vi "SetRotation.vi"(7 "Relative?":bool, 8 "error in (no error)":errorcluster, 9 "Angle":sgl, 10 "Axis":cluster{"X":sgl, "Y":sgl, "Z":sgl}={"X"=0.0, "Y"=1.0, "Z"=0.0}, 11 "3D Object in":refnum<class "3D Object.lvclass">) -> (0 "error out":errorcluster, 3 "3D Object out":refnum<class "3D Object.lvclass">)   [LabVIEW 2015, in "3D Object.lvclass"]
uses:
  3D Object.lvclass
  3D Object.lvclass/3D Object.ctl
  <vilib>/picture/3D Picture Control/NI_3D Picture Control.lvlib
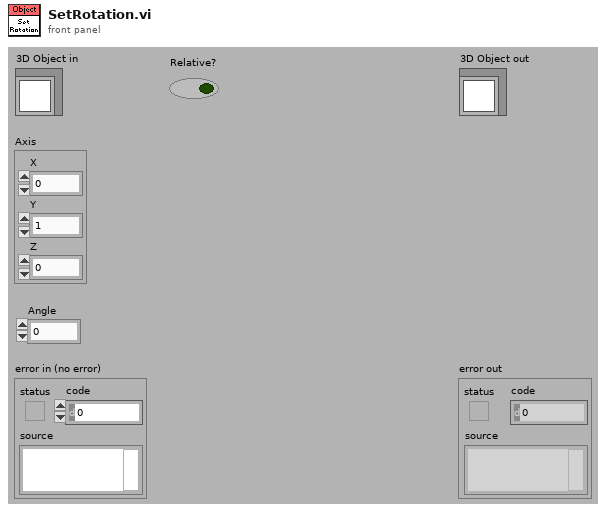
[diagram p1: front panel]
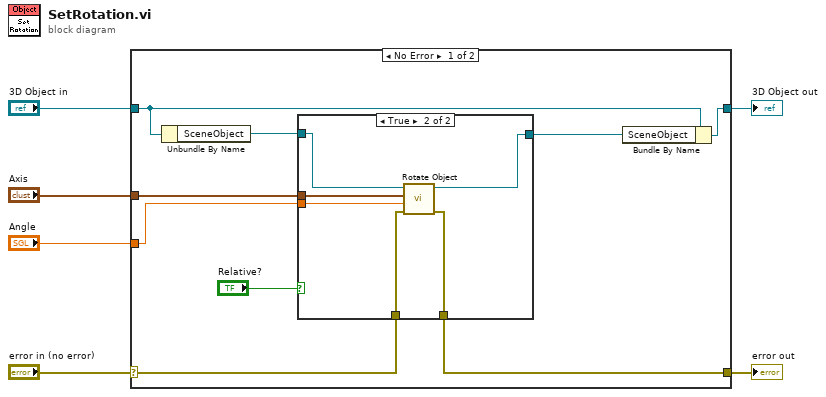
[diagram p0: block diagram]
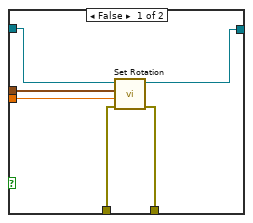
[diagram p2: hidden frame]
diagram:
  n1 = case shown="No Error" "error in (no error)" {
    selector: "error in (no error)" -> [w11 w29]
    tunnel: [w10 w29] -> w5
    tunnel: [w12 w28] -> w3
    tunnel: "3D Object in" -> [w13 w28]
    tunnel: "Angle" -> [w9 _]
    tunnel: "Axis" -> [w8 _]
    frame No Error {
      n2 = Unbundle By Name(w13) -> ("SceneObject"=w15:refnum<vi>)
      n3 = case shown="True" "Relative?" {
        tunnel: w15 -> [w21 w27]
        tunnel: [w20 w26] -> w14
        tunnel: w9 -> [w19 w25]
        tunnel: w11 -> [w18 w24]
        tunnel: [w17 w23] -> w10
        tunnel: w8 -> [w16 w22]
        frame False {
          n4 = call <vilib>:"Set Rotation.vi"("error in (no error)"=w18, "Angle"=w19, "Axis"=w16, "Scene Object"=w21) -> ("error out"=w17:errorcluster, "Rotated Scene Object"=w20:refnum<vi>)  [unwired: 6 out]
        }
        frame True {
          n5 = call <vilib>:"Rotate Object.vi"("error in (no error)"=w24, "Angle"=w25, "Axis"=w22, "Scene.Object In"=w27) -> ("error out"=w23:errorcluster, "Scene.Object Out"=w26:refnum<vi>)  [unwired: 6 out]
        }
      }
      n6 = Bundle By Name(cluster=w13, "SceneObject"=w14) -> (w12:refnum<class "3D Object.lvclass">)
    }
    frame Error {
    }
  }
  "error out" <- w5
  "3D Object out" <- w3
